vi "Untitled 1.vi"() -> ()   [LabVIEW 2015]
uses:
  Found Items.ctl
  JSONtext.lvlib
panel:
  out "Items":T1[](array[typedef])
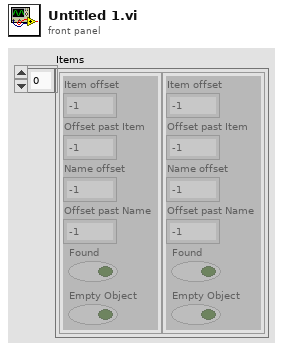
[diagram p1: front panel]
types:
  T1 = typedef "JSONtext.lvlib/Found Items.ctl" = cluster{"Item offset":i32, "Offset past Item":i32, "Name offset":i32, "Offset past Name":i32, "Found":bool, "Empty Object":bool}
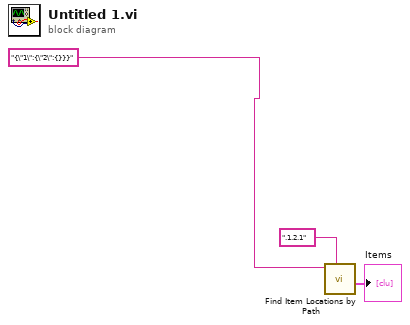
[diagram p0: block diagram]
diagram:
  n1 = call "Find Item Locations by Path.vi"("Path"=".1.2.1", "JSON"="{\"1\":{\"2\":{}}}") -> ("Items"=→"Items":T1[])  [unwired: 8 in, 1 out]
